vi "Buoyancy Force.vi"(10 "Height (m)":dbl, 11 "Density (kg/m^3)":dbl) -> (3 "Potential (Pa)":dbl)   [LabVIEW 2019]
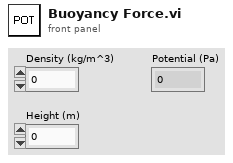
[diagram p1: front panel]
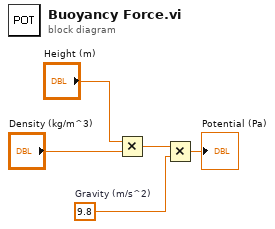
[diagram p0: block diagram]
diagram:
  w1 = 9.8  # Gravity (m/s^2)
  n1 = Multiply(x="Height (m)", y="Density (kg/m^3)") -> (x*y=w4:dbl)
  n2 = Multiply(x=w4, y=w1) -> (x*y=→"Potential (Pa)":dbl)
